vi "ZE_Recorder_ChannelConfigToString.vi"(8 "error in":errorcluster, 11 "channel config array":T1[](array[typedef])) -> (0 "error out":errorcluster, 3 "Config String":string)   [LabVIEW 2025, in "ZE_Recorder.lvlib"]
uses:
  ZE_Recorder.lvlib
  ZE_Recorder_TempConfigCluster.ctl
  ZE_Recorder_TempParam.ctl
  ZE_Recorder_TempType.ctl
  ZE_Recorder_TCCluster.ctl
  ZE_Recorder_TCSource.ctl
  ZE_Recorder_TCType.ctl
  ZE_Recorder_RTDCluster.ctl
panel:
  # "Connector Pane"
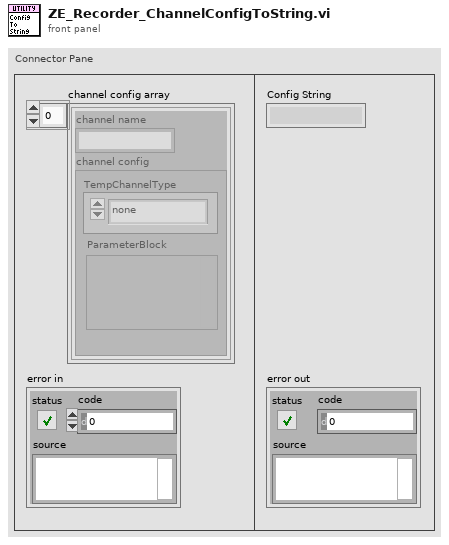
[diagram p1: front panel]
types:
  T1 = typedef "ZE_Recorder.lvlib/ZE_Recorder_TempConfigCluster.ctl" = cluster{"channel name":string, "channel config":T2}
  T2 = typedef "ZE_Recorder.lvlib/ZE_Recorder_TempParam.ctl" = cluster{"ParameterBlock":variant, "TempChannelType":T3}
  T3 = typedef "ZE_Recorder.lvlib/ZE_Recorder_TempType.ctl" = enum16{"none", "Thermocouple", "RTD", "Thermistor VE", "Thermistor CE"}
  T4 = typedef "ZE_Recorder.lvlib/ZE_Recorder_TCCluster.ctl" = cluster{"TC Cold Junction":dbl, "Cold Junction Source":T5, "TC Type":T6}
  T5 = typedef "ZE_Recorder.lvlib/ZE_Recorder_TCSource.ctl" = i32
  T6 = typedef "ZE_Recorder.lvlib/ZE_Recorder_TCType.ctl" = i32
  T7 = typedef "ZE_Recorder.lvlib/ZE_Recorder_RTDCluster.ctl" = cluster{"RTD R0":dbl, "RTD Iex":dbl, "RTD Type":i32, "RTD Config":i32}
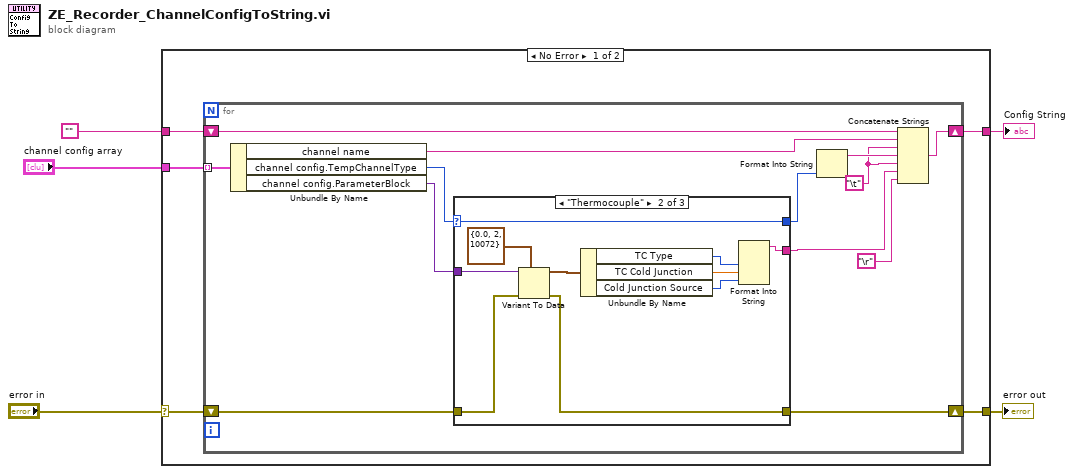
[diagram p0: block diagram]
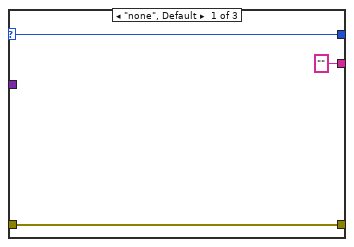
[diagram p2: hidden frame]
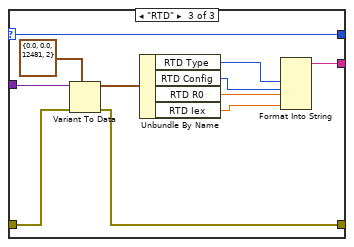
[diagram p3: hidden frame]
diagram:
  n1 = case shown="No Error" "error in" {
    selector: "error in" -> [w7 w48]
    tunnel: [w10 w49] -> w5
    tunnel: "" -> [w9 w49]
    tunnel: "channel config array" -> [w8 _]
    tunnel: [w6 w48] -> w1
    frame No Error {
      n2 = for {
        tunnel: w8 -> [w21] mode=indexing
        shift-right: [w22] -> w10
        shift-left: w9 -> [w23]
        shift-right: [w11] -> w6
        shift-left: w7 -> [w12]
        w18 = "\t"
        n3 = Unbundle By Name(w21) -> ("channel name"=w20:string, "channel config.TempChannelType"=w17:T3, "channel config.ParameterBlock"=w15:variant)
        n4 = case shown="\"Thermocouple\"" w17 {
          selector: w17 -> [w25 w36 w47]
          tunnel: [w25 w36 w47] -> w16
          tunnel: w15 -> [_ w35 w42]
          tunnel: ["" w27 w40] -> w14
          tunnel: w12 -> [w24 w33 w39]
          tunnel: [w24 w32 w38] -> w11
          frame "none", Default {
          }
          frame "Thermocouple" {
            n5 = Variant To Data(error in=w33, type=T4 {"TC Cold Junction"=0.0, "Cold Junction Source"=2, "TC Type"=10072} ("output cluster"), Variant=w35) -> (data=w34:T4, error out=w32:errorcluster)
            n6 = Unbundle By Name(w34) -> ("TC Type"=w30:T6, "TC Cold Junction"=w29:dbl, "Cold Junction Source"=w28:T5)
            n7 = Format Into String(w30, w29, w28) -> (resulting string=w27:string)  [unwired: 3 in, 1 out]
          }
          frame "RTD" {
            n8 = Variant To Data(error in=w39, type=T7 {"RTD R0"=0.0, "RTD Iex"=0.0, "RTD Type"=12481, "RTD Config"=2} ("RTD Config Cluster"), Variant=w42) -> (data=w46:T7, error out=w38:errorcluster)
            n9 = Unbundle By Name(w46) -> ("RTD Type"=w45:i32, "RTD Config"=w44:i32, "RTD R0"=w43:dbl, "RTD Iex"=w41:dbl)
            n10 = Format Into String(w45, w44, w43, w41) -> (resulting string=w40:string)  [unwired: 3 in, 1 out]
          }
        }
        n11 = Format Into String(w16) -> (resulting string=w19:string)  [unwired: 3 in, 1 out]
        n12 = Concatenate Strings(w23, w20, w18, w19, w18, w14, "\r") -> (w22:string)
      }
    }
    frame Error {
    }
  }
  "Config String" <- w5
  "error out" <- w1
